vi "Configuration 1.1 Initialize.vi"(8 "error in (no error)":errorcluster, 10 "dsf version":T2, 11 "dsf configuration json":string) -> (0 "error out":errorcluster, 3 "framework configuration 1.1":T1={"plugins"=[{"name"="Plugin", "components"=[], "cycle timing"={"priority"=10000, "decimation"=1, "offset"=0}, "threads"=[], "transfer groups"=[{"name"="Group", "direction"=0, "cycle timing"={"priority"=100, "decimation"=1, "offset"=0}, "thread index"=-1, "settings"=[], "transfers"=[{"name"="Transfer", "byte order"=0, "settings"=[], "channels"=[{"string offset"=0, "string data type"=2, "engine data type"=2, "name"="Channel", "settings"=[], "units"="V"}]}], "timeout behavior"=0}], "settings"=[]}]})   [LabVIEW 2019, in "DSF Core.lvlib" / "Configuration Session.lvclass"]
uses:
  Configuration Session.lvclass
  Typedefs/DSF Version Info.ctl
  DSF Core.lvlib
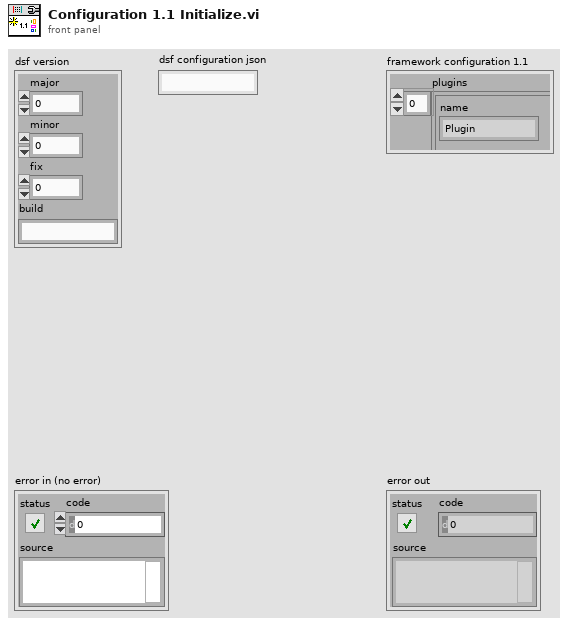
[diagram p1: front panel]
types:
  T1 = cluster{"plugins":cluster{"name":string, "components":string[], "cycle timing":cluster{"priority":u64, "decimation":u64, "offset":u64}, "threads":cluster{"buffer converter settings":cluster{"key":string, "value":string}[], "transceiver settings":cluster{"key":string, "value":string}[], "custom settings":cluster{"key":string, "value":string}[], "processor":i32, "priority offset":i16}[], "transfer groups":cluster{"name":string, "direction":u8, "cycle timing":cluster{"priority":u64, "decimation":u64, "offset":u64}, "thread index":i32, "settings":cluster{"key":string, "value":string}[], "transfers":cluster{"name":string, "byte order":u8, "settings":cluster{"key":string, "value":string}[], "channels":cluster{"string offset":u64, "string data type":u8, "engine data type":u8, "name":string, "settings":cluster{"key":string, "value":string}[], "units":string}[]}[], "timeout behavior":u8}[], "settings":cluster{"key":string, "value":string}[]}[]}
  T2 = typedef "DSF Core.lvlib/DSF Version Info.ctl" = cluster{"major":u32, "minor":u32, "fix":u32, "build":string}
  T3 = cluster{"plugins":cluster{"id":string, "values":cluster{"components":string[], "timing":cluster{"priority":u64, "decimation":u64, "offset":u64}, "group ids":string[], "settings id":string, "threads":cluster{"buffer converter settings":cluster{"key":string, "value":string}[], "transceiver settings":cluster{"key":string, "value":string}[], "custom settings":cluster{"key":string, "value":string}[], "processor":i32, "priority offset":i16}[]}}[], "groups":cluster{"id":string, "values":cluster{"direction":i32, "timing":cluster{"priority":u64, "decimation":u64, "offset":u64}, "transfer ids":string[], "settings id":string, "thread":i32, "timeout behavior":u8}}[], "transfers":cluster{"id":string, "values":cluster{"byte order":i32, "channel ids":string[], "settings id":string}}[], "channels":cluster{"id":string, "values":cluster{"string buffer offset":u64, "string data type":i32, "engine data type":i32, "settings id":string, "units":string}}[], "settings":cluster{"id":string, "values":cluster{"key":string, "value":string}[]}[]}
  T4 = cluster{"Plugins":cluster{"name":string, "components":string[], "cycle timing":cluster{"priority":u64, "decimation":u64, "offset":u64}, "threads":cluster{"buffer converter settings":cluster{"key":string, "value":string}[], "transceiver settings":cluster{"key":string, "value":string}[], "custom settings":cluster{"key":string, "value":string}[], "processor":i32, "priority offset":i16}[], "Transfer Groups":cluster{"name":string, "direction":enum8{"Tx", "Rx"}, "cycle timing":cluster{"priority":u64, "decimation":u64, "offset":u64}, "thread index":i32, "settings":cluster{"key":string, "value":string}[], "Transfers":cluster{"name":string, "byte order":enum8{"big-endian", "little-endian"}, "settings":cluster{"key":string, "value":string}[], "channels":cluster{"string offset":u64, "string data type":enum8{"Bool", "SGL", "DBL", "I8", "I16", "I32", "I64", "U8", "U16", "U32", "U64"}, "engine data type":enum8{"Bool", "SGL", "DBL", "I8", "I16", "I32", "I64", "U8", "U16", "U32", "U64"}, "name":string, "settings":cluster{"key":string, "value":string}[], "units":string}[]}[], "timeout behavior":enum8{"Increment Late Count", "Throw Error"}}[], "settings":cluster{"key":string, "value":string}[]}[]}
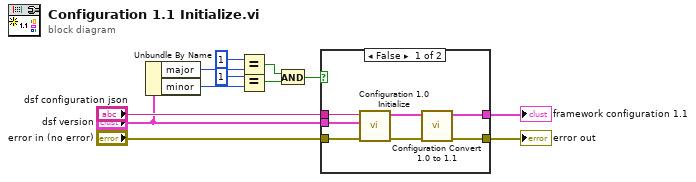
[diagram p0: block diagram]
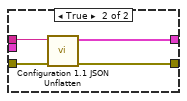
[diagram p2: hidden frame]
diagram:
  n1 = Unbundle By Name("dsf version") -> ("major"=w8:u32, "minor"=w11:u32)
  n2 = Equal?(x=u32 1, y=w8) -> (x = y?=w4:bool)
  n3 = Equal?(x=u32 1, y=w11) -> (x = y?=w5:bool)
  n4 = And(x=w4, y=w5) -> (x .and. y?=w3:bool)
  n5 = case shown="False" w3 {
    tunnel: "error in (no error)" -> [w18 w23]
    tunnel: "dsf configuration json" -> [w19 w22]
    tunnel: [w14 w21] -> w10
    tunnel: [w15 w20] -> w9
    tunnel: "dsf version" -> [w13 _]
    frame False {
      n6 = call "Configuration 1.0 Initialize.vi"("error in (no error)"=w18, "dsf version"=w13, "dsf configuration json"=w19) -> ("error out"=w17:errorcluster, "framework configuration 1.0"=w16:T3)  [unwired: 7 in]
      n7 = call "Configuration Convert 1.0 to 1.1.vi"("error in (no error)"=w17, "framework configuration 1.0"=w16) -> ("error out"=w15:errorcluster, "framework configuration 1.1"=w14:T4)  [unwired: 8 in]
    }
    frame True {
      n8 = call "Configuration 1.1 JSON Unflatten.vi"("error in (no error)"=w23, "dsf configuration json"=w22) -> ("error out"=w20:errorcluster, "framework configuration 1.1"=w21:T1)  [unwired: 8 in]
    }
  }
  "error out" <- w9
  "framework configuration 1.1" <- w10
